vi "Run.vi"(8 "error in (no error)":errorcluster, 9 "Time Ratio used":dbl, 10 "Maze (0: Empty, -1: Enemy. >0: Teammate":i32[][](array[numeric]), 11 "TeamEffort in":refnum<class "TeamEffort.lvclass">) -> (0 "error out":errorcluster, 1 "Direction":T1, 2 "Action":T2, 3 "TeamEffort out":refnum<class "TeamEffort.lvclass">, 4 "Replicated":refnum<class "Square.lvclass">)   [LabVIEW 2015, in "TeamEffort.lvclass"]
uses:
  TeamEffort.lvclass
  Type Defs/Action Enum.ctl
  Type Defs/Direction Enum.ctl
  Square/Square.lvclass
  TeamEffort.lvclass/TeamEffort.ctl
panel:
  # "NOTICE - YOU MUST NOT REMOVE THIS NOTICE. PER THE FOLLOWING LICENSE, YOU MAY REPRODUCE THIS SOFTWARE PROVIDED YOU FOLLOW THE TERMS\nOF THE LICENSE.\n\n---BEGIN BSD LICENSE (http://opensource.org/licenses/BSD-2-Clause)---\nCopyright (c) 2015, Endigit, Inc. <robert@endigit.com>\nAll rights reserved.\n\nRedistribution and use in source and binary forms, with or without modification, are permitted provided that the following conditions are met:\n\n1. Redistributions of source code must retain the above copyright notice, this list of conditions and the following disclaimer.\n\n2. Redistributions in binary form must reproduce the above copyright notice, this list of conditions and the following disclaimer in the documentation and/or other \nmaterials provided with the distribution.\n\nTHIS SOFTWARE IS PROVIDED BY THE COPYRIGHT HOLDERS AND CONTRIBUTORS \"AS IS\" AND ANY EXPRESS OR IMPLIED WARRANTIES, INCLUDING, BUT NOT \nLIMITED TO, THE IMPLIED WARRANTIES OF MERCHANTABILITY AND FITNESS FOR A PARTICULAR PURPOSE ARE DISCLAIMED. IN NO EVENT SHALL THE COPYRIGHT \nHOLDER OR CONTRIBUTORS BE LIABLE FOR ANY DIRECT, INDIRECT, INCIDENTAL, SPECIAL, EXEMPLARY, OR CONSEQUENTIAL DAMAGES (INCLUDING, BUT NOT \nLIMITED TO, PROCUREMENT OF SUBSTITUTE GOODS OR SERVICES; LOSS OF USE, DATA, OR PROFITS; OR BUSINESS INTERRUPTION) HOWEVER CAUSED AND ON \nANY THEORY OF LIABILITY, WHETHER IN CONTRACT, STRICT LIABILITY, OR TORT (INCLUDING NEGLIGENCE OR OTHERWISE) ARISING IN ANY WAY OUT OF THE USE \nOF THIS SOFTWARE, EVEN IF ADVISED OF THE POSSIBILITY OF SUCH DAMAGE.\n---END BSD LICENSE---"
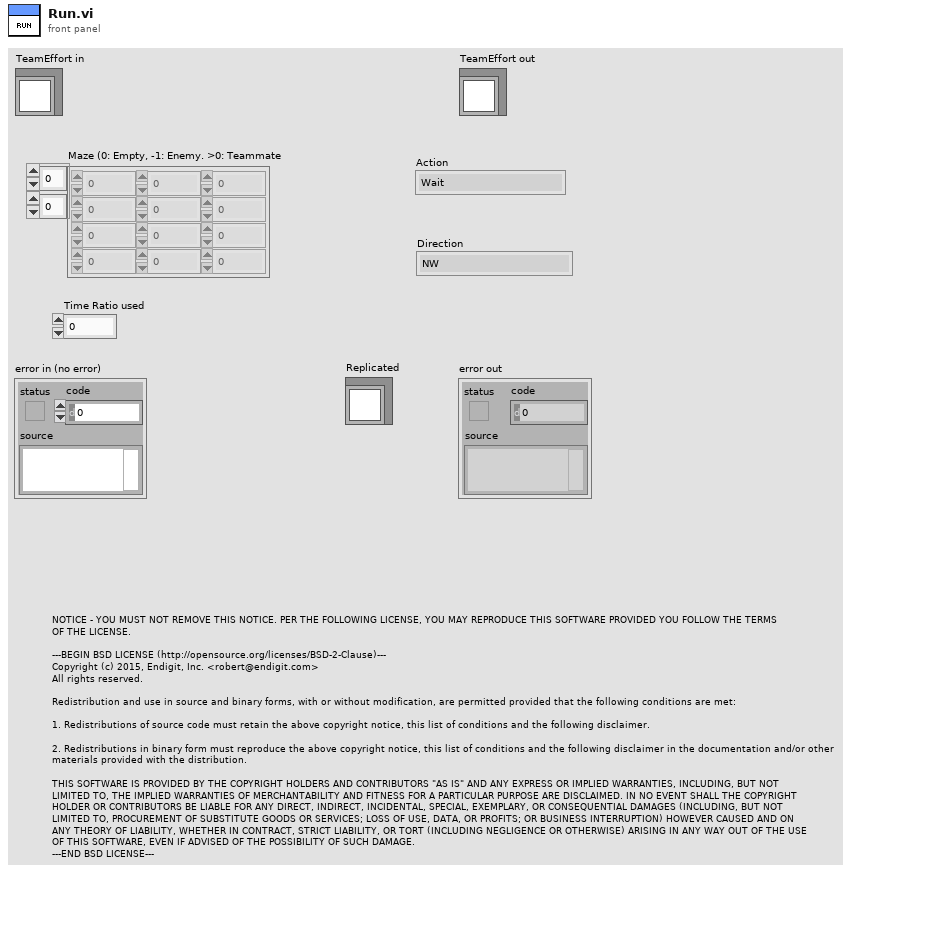
[diagram p1: front panel]
types:
  T1 = typedef "Square.lvclass/Direction Enum.ctl" = enum16{"NW", "N", "NE", "E", "SE", "S", "SW", "W"}
  T2 = typedef "Square.lvclass/Action Enum.ctl" = enum16{"Wait", "Move", "Attack", "Replicate"}
  T3 = typedef "TeamEffort.lvclass/Grid Cluster.ctl" = cluster{"p[x][y]":i32[][], "Move Count":i32, "Info[p]":T4[]}
  T4 = typedef "TeamEffort.lvclass/Player Cluster.ctl" = cluster{"Player #":i32, "Exp. Move":i32, "X":i16, "Y":i16, "Action":T2, "Direction":T1, "Moved?":bool, "Replicated":refnum<class "Square.lvclass">}
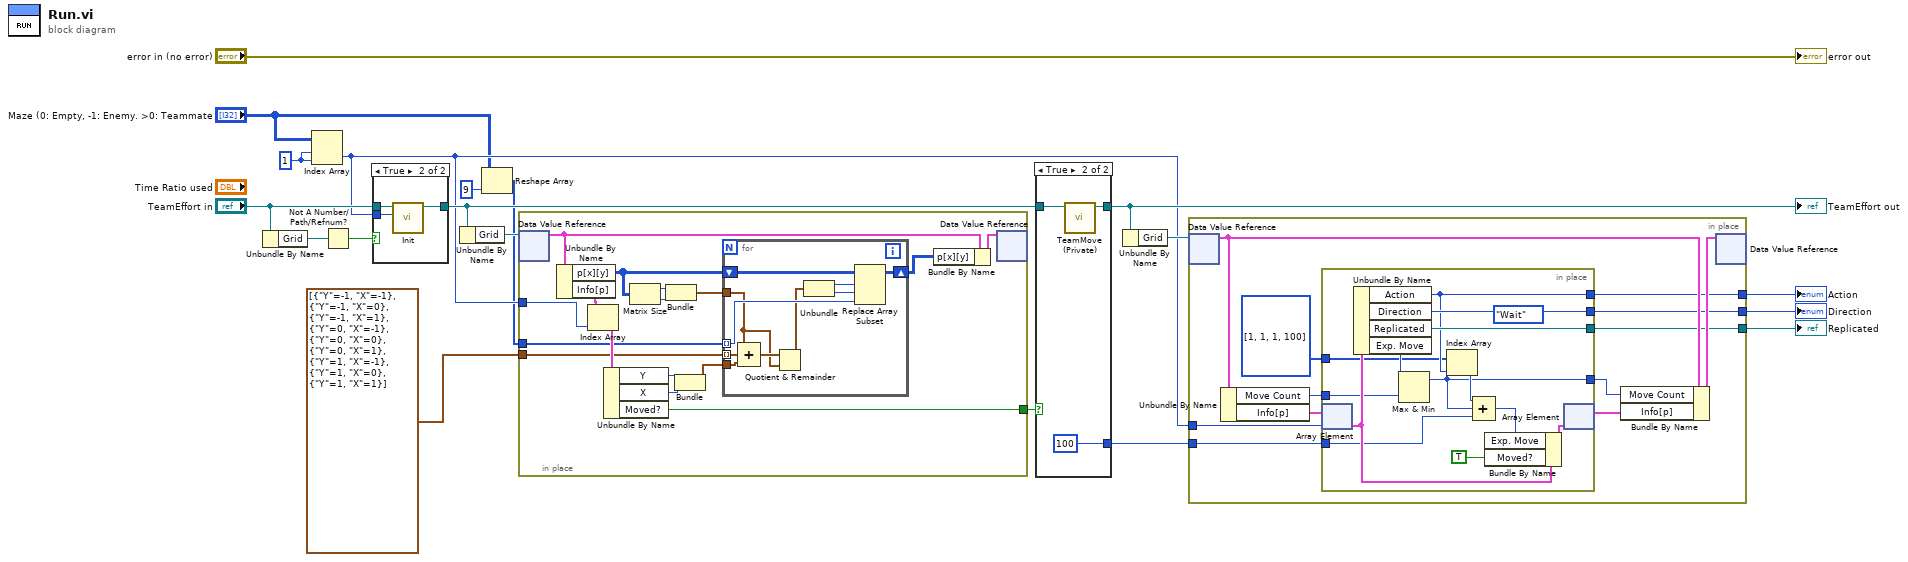
[diagram p0: block diagram]
diagram:
  w16 = 1
  n1 = Unbundle By Name("TeamEffort in") -> ("Grid"=w19:refnum<data-value>)
  n2 = Index Array(array="Maze (0: Empty, -1: Enemy. >0: Teammate", index (row)=w16, index (col)=w16) -> (element=w9:i32)
  n3 = Not A Number/Path/Refnum?(number/path/refnum=w19) -> (NaN/Path/Refnum?=w13:bool)
  n4 = case shown="True" w13 {
    tunnel: "TeamEffort in" -> [w20 w23]
    tunnel: [w20 w22] -> w14
    tunnel: w9 -> [_ w21]
    frame False {
    }
    frame True {
      n5 = call-dynamic "Init.vi"("Player ID"=w21, "TeamEffort in"=w23) -> ("TeamEffort out"=w22:refnum<class "TeamEffort.lvclass">)  [unwired: 9 in]
    }
  }
  n6 = Unbundle By Name(w14) -> ("Grid"=w17:refnum<data-value>)
  n7 = Reshape Array("Maze (0: Empty, -1: Enemy. >0: Teammate", 9 ("dimension size")) -> (w6:i32[])
  n8 = in-place {
    in-place-border: w9 -> [w39]
    in-place-border: [w35] -> w12
    in-place-border: w6 -> [w32]
    in-place-border: cluster{"Y":i32, "X":i32}[] [{"Y"=-1, "X"=-1}, {"Y"=-1, "X"=0}, {"Y"=-1, "X"=1}, {"Y"=0, "X"=-1}, {"Y"=0, "X"=0}, {"Y"=0, "X"=1}, {"Y"=1, "X"=-1}, {"Y"=1, "X"=0}, {"Y"=1, "X"=1}] -> [w33]
    n9 = in-place-dvr #1(w17) -> (w36:T3)  [unwired: 1 out]
    n10 = Unbundle By Name(w36) -> ("p[x][y]"=w28:i32[][], "Info[p]"=w38:T4[])
    n11 = Index Array(array=w38, index=w39) -> (element=w37:T4)
    n12 = Unbundle By Name(w37) -> ("Y"=w31:i16, "X"=w30:i16, "Moved?"=w35:bool)
    n13 = Matrix Size(0:w28) -> (1:w27:i32, 2:w26:i32)
    n14 = Bundle("number of columns"=w27, "matrix"=w26) -> (w25:cluster{"number of columns":i32, "matrix":i32})  [unwired: 1 in]
    n15 = Bundle("Y"=w31, "X"=w30) -> (w29:cluster{"Y":i16, "X":i16})  [unwired: 1 in]
    n16 = for {
      shift-right: [w48] -> w24
      shift-left: w28 -> [w49]
      tunnel: w33 -> [w47] mode=indexing
      tunnel: w32 -> [w45] mode=indexing
      tunnel: w29 -> [w46]
      tunnel: w25 -> [w43]
      n17 = Compound Arithmetic op=ADD(w43, w47, w46) -> (w44:cluster{i32, i32})
      n18 = Quotient & Remainder(x=w44, y=w43) -> (x-y*floor(x/y)=w42:cluster{i32, i32})  [unwired: 1 out]
      n19 = Unbundle(w42) -> (w41:i32, w40:i32)
      n20 = Replace Array Subset(array=w49, new element=w45, index (row)=w41, index (col)=w40) -> (w48:i32[][])
    }
    n21 = Bundle By Name(cluster=w36, "p[x][y]"=w24) -> (w34:T3)
    n22 = in-place-dvr #1(w34) -> ()  [unwired: 2 out]
  }
  n23 = case shown="True" w12 {
    tunnel: [w50 w53] -> w11
    tunnel: w14 -> [w50 w52]
    tunnel: [_ 100] -> w1
    frame False {
    }
    frame True {
      n24 = call "TeamMove (Private).vi"("TeamEffort in"=w52) -> ("TeamEffort out"=w53:refnum<class "TeamEffort.lvclass">)  [unwired: 9 in, 1 out]
    }
  }
  "TeamEffort out" <- w11
  n25 = Unbundle By Name(w11) -> ("Grid"=w10:refnum<data-value>)
  n26 = in-place {
    in-place-border: w9 -> [w62]
    in-place-border: [w60] -> w4
    in-place-border: [w59] -> w3
    in-place-border: [w58] -> w2
    in-place-border: w1 -> [w54]
    n27 = in-place-dvr #2(w10) -> (w65:T3)  [unwired: 1 out]
    n28 = Unbundle By Name(w65) -> ("Move Count"=w57:i32, "Info[p]"=w63:T4[])
    n29 = in-place {
      in-place-border: [w71] -> w60
      in-place-border: [w75] -> w59
      in-place-border: [w74] -> w58
      in-place-border: w57 -> [w72]
      in-place-border: [w68] -> w56
      in-place-border: i32[] [1, 1, 1, 100] -> [w70]
      in-place-border: w54 -> [w66]
      (unwired) Action_Enum."Wait" ("Action")
      n30 = in-place-array #3(w63, w62) -> (w76:T4)
      n31 = Unbundle By Name(w76) -> ("Action"=w71:T2, "Direction"=w75:T1, "Replicated"=w74:refnum<class "Square.lvclass">, "Exp. Move"=w73:i32)
      n32 = Max & Min(x=w73, y=w72) -> (max(x,y)=w68:i32)  [unwired: 1 out]
      n33 = Index Array(array=w70, index=w71) -> (element=w69:i32)
      n34 = Compound Arithmetic op=ADD(w69, w68, w66) -> (w67:i32)
      n35 = Bundle By Name(cluster=w76, "Exp. Move"=w67, "Moved?"=TRUE) -> (w77:T4)
      n36 = in-place-array #3(w77) -> (w61:T4[])  [unwired: 1 out]
    }
    n37 = Bundle By Name(cluster=w65, "Move Count"=w56, "Info[p]"=w61) -> (w64:T3)
    n38 = in-place-dvr #2(w64) -> ()  [unwired: 2 out]
  }
  "Action" <- w4
  "Direction" <- w3
  "Replicated" <- w2
  "error out" <- "error in (no error)"
